vi "Open Subpanel UI Reference.vi"(0 "Controller in":refnum<class "Generic Plugin.lvclass">, 1 "error in (no error)":errorcluster) -> (2 "Controller out":refnum<class "Generic Plugin.lvclass">, 3 "vi reference":refnum<vi>, 4 "error out":errorcluster)   [LabVIEW 2020, in "Generic Plugin.lvclass"]
doc: "Get a reference for the Subpanel UI.vi of the controller."
uses:
  Generic Plugin.lvclass
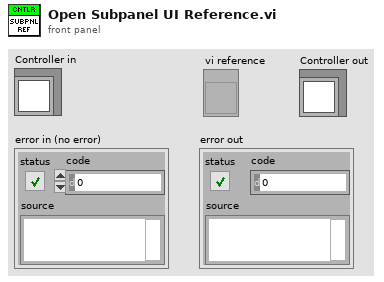
[diagram p1: front panel]
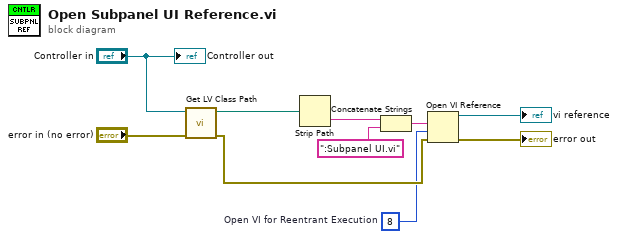
[diagram p0: block diagram]
diagram:
  w1 = 8  # Open VI for Reentrant Execution
  n1 = call <vilib>:"Get LV Class Path.vi"("error in (no error)"="error in (no error)", "object"="Controller in") -> ("error out"=w10:errorcluster, "class path"=w4:path)  [unwired: 8 in]
  n2 = Strip Path(path=w4) -> (name=w5:string)  [unwired: 1 out]
  n3 = Concatenate Strings(w5, ":Subpanel UI.vi" ("string")) -> (w7:string)
  n4 = Open VI Reference(vi path=w7, options=w1, error in (no error)=w10) -> (vi reference=→"vi reference":refnum<vi>, error out=→"error out":errorcluster)  [unwired: 3 in]
  "Controller out" <- "Controller in"
